vi "Generic Parser.vi"(8 "Error In":errorcluster, 9 "Measurement List In":string, 10 "Data Array In":dbl[](array[numeric])) -> (0 "Error Out":errorcluster, 2 "Waveform Measurement Out":dynamicdata(graph))   [LabVIEW 2013, in "Generic Instrument.lvlib" / "Generic Instrument.lvclass"]
doc: "This VI takes any measurent Array of Strings and accompanying measurement Array fo Numbers and put them in a waveform format."
uses:
  Generic Instrument.lvclass
  Data Logger/Data Logger.lvclass
panel:
  out "Numeric":dbl
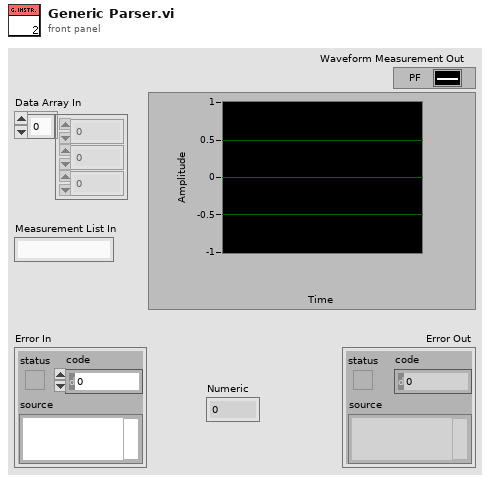
[diagram p1: front panel]
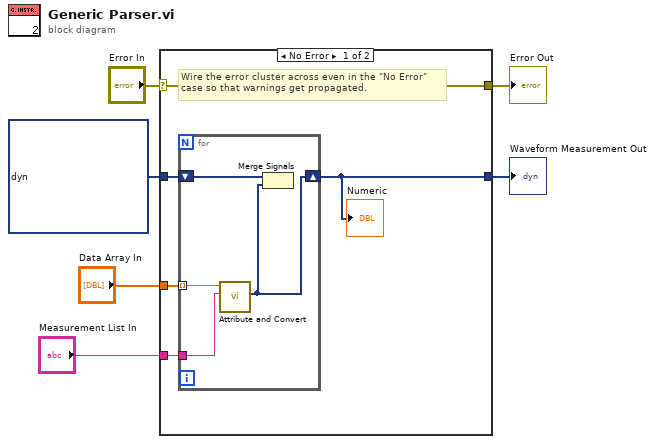
[diagram p0: block diagram]
diagram:
  n1 = case shown="No Error" "Error In" {
    selector: "Error In" -> [w11 w17]
    tunnel: [w11 w17] -> w5
    tunnel: "Data Array In" -> [w10 _]
    tunnel: "Measurement List In" -> [w9 _]
    tunnel: dynamicdata [] ("Waveform Graph 2") -> [w8 w16]
    tunnel: [w7 w16] -> w1
    frame No Error {
      # "Wire the error cluster across even in the \"No Error\"\ncase so that warnings get propagated."
      n2 = for {
        tunnel: w10 -> [w15] mode=indexing
        tunnel: w9 -> [w14]
        shift-right: [w12] -> w7
        shift-left: w8 -> [w13]
        n3 = call "Attribute and Convert.vi"("Signal Name"=w14, "Number in"=w15) -> ("Dynamic Signal Out"=w12:dynamicdata)  [unwired: 9 in]
        n4 = Merge Signals(w13, w12) -> ()  [unwired: 1 out]
      }
      "Numeric" <- w7
    }
    frame Error {
    }
  }
  "Error Out" <- w5
  "Waveform Measurement Out" <- w1
